vi "数据存储接口.vi"(4 "快捷测试？":bool, 5 "质控参数设置":T1, 6 "标样校准？":bool, 7 "数据标记表":string, 8 "空白校准？":bool, 10 "数据存储模式":T2(ring), 11 "测量数据区":T4) -> (3 "data输出":T3)   [LabVIEW 2016, in "斯坦道总氮.lvlib"]
panel:
  # "跨度值"
  # "零点核查标准液浓度"
  # "跨度核查标准液浓度"
  # "标样核查标准液浓度"
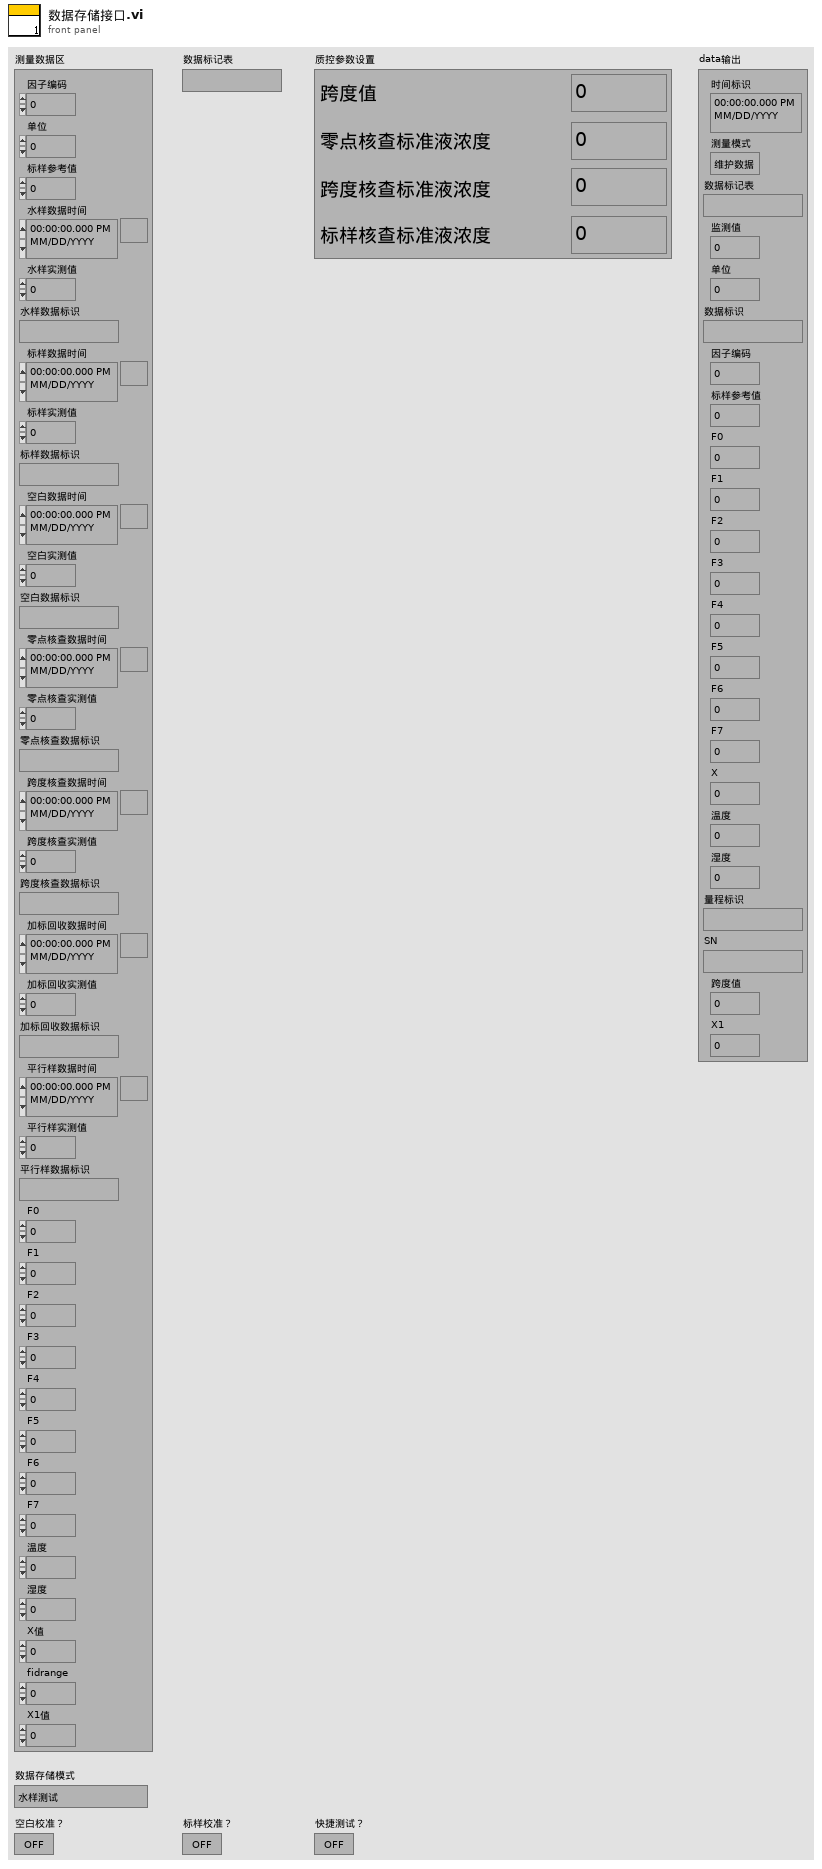
[diagram p1: front panel]
types:
  T1 = cluster{"跨度值":dbl, "零点标准液浓度":dbl, "跨度标准液浓度":dbl, "标准液标准浓度":dbl}
  T2 = enum16{"水样测试", "标样核查", "跨度核查", "零点核查", "加标回收", "空白测试", "平行样"}
  T3 = cluster{"时间标识":timestamp, "测量模式":enum16{"维护数据", "水样测试", "标样核查", "零点核查", "跨度核查", "空白测试", "平行样测试", "加标回收", "空白校准", "标样校准", "初始化（清洗）", "快捷测试"}, "数据标记表":string, "监测值":sgl, "单位":u16, "数据标识":string, "因子编码":u32, "标样参考值":sgl, "F0":sgl, "F1":sgl, "F2":sgl, "F3":sgl, "F4":sgl, "F5":sgl, "F6":sgl, "F7":sgl, "X":sgl, "温度":sgl, "湿度":sgl, "量程标识":string, "SN":string, "跨度值":sgl, "X1":sgl}
  T4 = cluster{"因子编码":u32, "单位":u16, "标样参考值":sgl, "水样数据时间":timestamp, "水样实测值":sgl, "水样数据标识":string, "标样数据时间":timestamp, "标样实测值":sgl, "标样数据标识":string, "空白数据时间":timestamp, "空白实测值":sgl, "空白数据标识":string, "零点核查数据时间":timestamp, "零点核查实测值":sgl, "零点核查数据标识":string, "跨度核查数据时间":timestamp, "跨度核查实测值":sgl, "跨度核查数据标识":string, "加标回收数据时间":timestamp, "加标回收实测值":sgl, "加标回收数据标识":string, "平行样数据时间":timestamp, "平行样实测值":sgl, "平行样数据标识":string, "F0":sgl, "F1":sgl, "F2":sgl, "F3":sgl, "F4":sgl, "F5":sgl, "F6":sgl, "F7":sgl, "温度":sgl, "湿度":sgl, "X值":sgl, "fidrange":u16, "X1值":sgl}
  T5 = enum16{"维护数据", "水样测试", "标样核查", "零点核查", "跨度核查", "空白测试", "平行样测试", "加标回收", "空白校准", "标样校准", "初始化（清洗）", "快捷测试"}
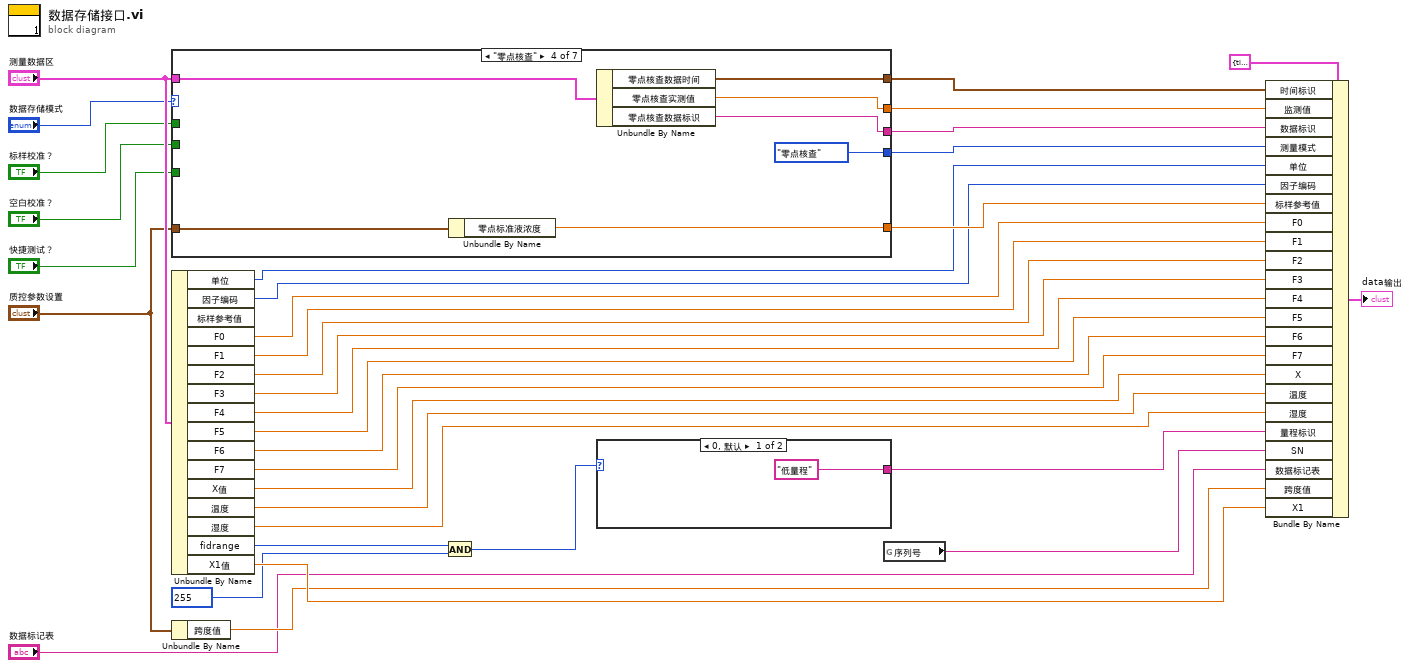
[diagram p0: block diagram]
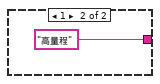
[diagram p2: hidden frame]
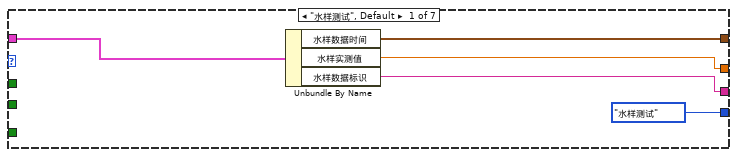
[diagram p3: hidden frame]
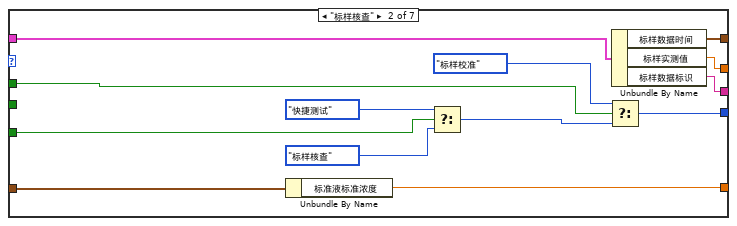
[diagram p4: hidden frame]
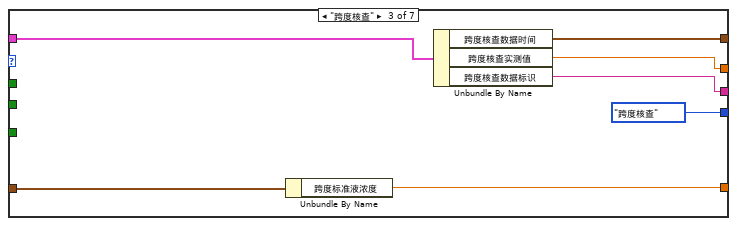
[diagram p5: hidden frame]
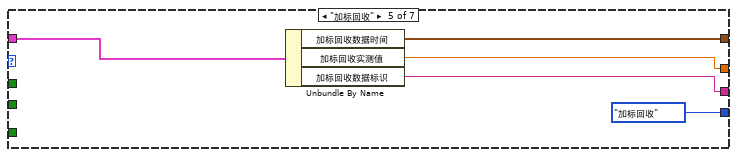
[diagram p6: hidden frame]
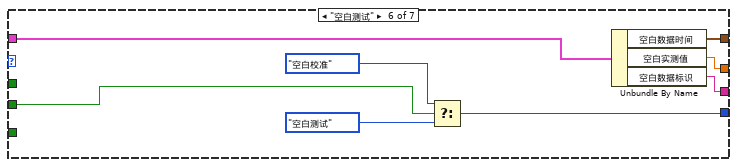
[diagram p7: hidden frame]
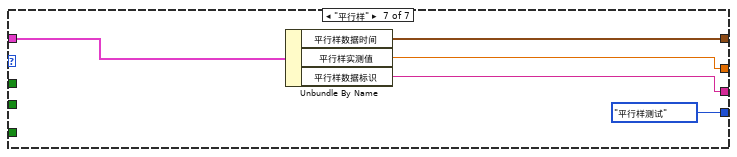
[diagram p8: hidden frame]
diagram:
  n1 = case shown="\"零点核查\"" "数据存储模式" {
    tunnel: "测量数据区" -> [w39 w52 w59 w66 w71 w79 w84]
    tunnel: [w38 w51 w58 w65 w70 w78 w83] -> w20
    tunnel: [w37 w50 w57 w64 w69 w77 w82] -> w19
    tunnel: [w36 w49 w56 w63 w68 w76 w81] -> w18
    tunnel: [T5."水样测试" ("测量模式") w42 T5."跨度核查" ("测量模式") T5."零点核查" ("测量模式") T5."加标回收" ("测量模式") w73 T5."平行样测试" ("测量模式")] -> w30
    tunnel: "质控参数设置" -> [_ w48 w55 w62 _ _ _]
    tunnel: [_ w47 w54 w61 _ _ _] -> w22
    tunnel: "空白校准？" -> [_ _ _ _ _ w72 _]
    tunnel: "标样校准？" -> [_ w41 _ _ _ _ _]
    tunnel: "快捷测试？" -> [_ w40 _ _ _ _ _]
    frame "水样测试", Default {
      n2 = Unbundle By Name(w39) -> ("水样数据时间"=w38:timestamp, "水样实测值"=w37:sgl, "水样数据标识"=w36:string)
    }
    frame "标样核查" {
      n3 = Unbundle By Name(w48) -> ("标准液标准浓度"=w47:dbl)
      n4 = Select(t=T5."快捷测试" ("测量模式"), s=w40, f=T5."标样核查" ("测量模式")) -> (s? t:f=w43:T5)
      n5 = Select(t=T5."标样校准" ("测量模式"), s=w41, f=w43) -> (s? t:f=w42:T5)
      n6 = Unbundle By Name(w52) -> ("标样数据时间"=w51:timestamp, "标样实测值"=w50:sgl, "标样数据标识"=w49:string)
    }
    frame "跨度核查" {
      n7 = Unbundle By Name(w55) -> ("跨度标准液浓度"=w54:dbl)
      n8 = Unbundle By Name(w59) -> ("跨度核查数据时间"=w58:timestamp, "跨度核查实测值"=w57:sgl, "跨度核查数据标识"=w56:string)
    }
    frame "零点核查" {
      n9 = Unbundle By Name(w62) -> ("零点标准液浓度"=w61:dbl)
      n10 = Unbundle By Name(w66) -> ("零点核查数据时间"=w65:timestamp, "零点核查实测值"=w64:sgl, "零点核查数据标识"=w63:string)
    }
    frame "加标回收" {
      n11 = Unbundle By Name(w71) -> ("加标回收数据时间"=w70:timestamp, "加标回收实测值"=w69:sgl, "加标回收数据标识"=w68:string)
    }
    frame "空白测试" {
      n12 = Select(t=T5."空白校准" ("测量模式"), s=w72, f=T5."空白测试" ("测量模式")) -> (s? t:f=w73:T5)
      n13 = Unbundle By Name(w79) -> ("空白数据时间"=w78:timestamp, "空白实测值"=w77:sgl, "空白数据标识"=w76:string)
    }
    frame "平行样" {
      n14 = Unbundle By Name(w84) -> ("平行样数据时间"=w83:timestamp, "平行样实测值"=w82:sgl, "平行样数据标识"=w81:string)
    }
  }
  n15 = Unbundle By Name("测量数据区") -> ("单位"=w5:u16, "因子编码"=w6:u32, "F0"=w7:sgl, "F1"=w8:sgl, "F2"=w9:sgl, "F3"=w10:sgl, "F4"=w11:sgl, "F5"=w12:sgl, "F6"=w13:sgl, "F7"=w14:sgl, "X值"=w15:sgl, "温度"=w16:sgl, "湿度"=w17:sgl, "fidrange"=w23:u16, "X1值"=w34:sgl)  [unwired: 1 out]
  n16 = Unbundle By Name("质控参数设置") -> ("跨度值"=w32:dbl)
  n17 = And(x=w23, y=u16 255) -> (x .and. y?=w25:u16)
  n18 = case shown="0, 默认" w25 {
    tunnel: ["低量程" ("格式字符串") "高量程" ("格式字符串")] -> w26
    frame 0, Default {
    }
    frame 1 {
    }
  }
  n19 = global read "VAR总磷总氮全局变量.vi" "序列号"() -> (w28:string)
  n20 = Bundle By Name(cluster=T3 {"时间标识"=timestamp(0 s since 1904-01-01), "测量模式"=enum."维护数据", "数据标记表"="", "监测值"=0.0, "单位"=0, "数据标识"="", "因子编码"=0, "标样参考值"=0.0, "F0"=0.0, "F1"=0.0, "F2"=0.0, "F3"=0.0, "F4"=0.0, "F5"=0.0, "F6"=0.0, "F7"=0.0, "X"=0.0, "温度"=0.0, "湿度"=0.0, "量程标识"="", "SN"="", "跨度值"=0.0, "X1"=0.0} ("data输入"), "时间标识"=w20, "监测值"=w19, "数据标识"=w18, "测量模式"=w30, "单位"=w5, "因子编码"=w6, "标样参考值"=w22, "F0"=w7, "F1"=w8, "F2"=w9, "F3"=w10, "F4"=w11, "F5"=w12, "F6"=w13, "F7"=w14, "X"=w15, "温度"=w16, "湿度"=w17, "量程标识"=w26, "SN"=w28, "数据标记表"="数据标记表", "跨度值"=w32, "X1"=w34) -> (→"data输出":T3)
